vi "Close.vi"(8 "error in (no error)":errorcluster, 11 "RemoteConnection in":refnum<class "RemoteConnection.lvclass">) -> (0 "error out":errorcluster, 3 "RemoteConnection out":refnum<class "RemoteConnection.lvclass">)   [LabVIEW 2013, in "RemoteConnection.lvclass"]
uses:
  RemoteConnection.lvclass
  RemoteConnection.lvclass/RemoteConnection.ctl
  Message/VariantMessage/VariantMessage.lvclass
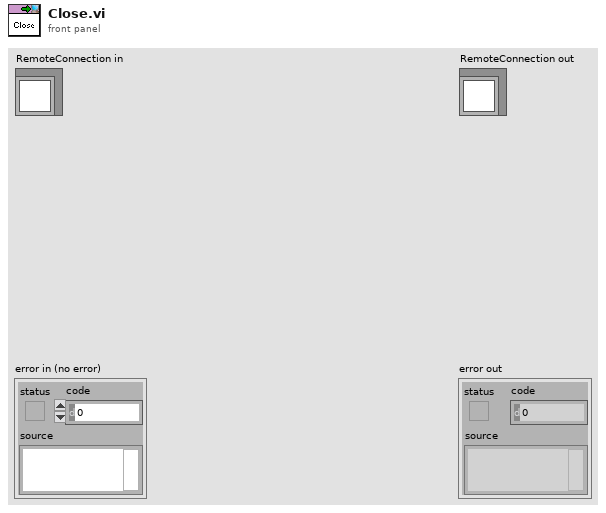
[diagram p1: front panel]
types:
  T1 = typedef "message_queue.ctl" = refnum<queue>
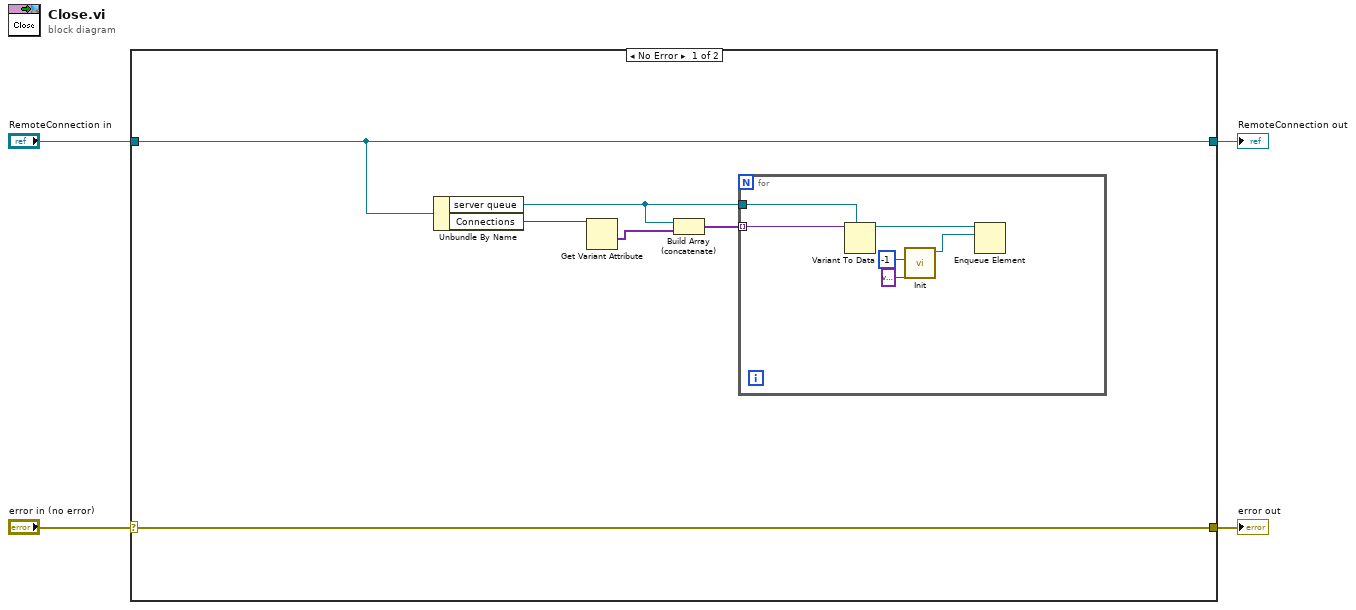
[diagram p0: block diagram]
diagram:
  n1 = case shown="No Error" "error in (no error)" {
    selector: "error in (no error)" -> [w10 w18]
    tunnel: [w10 w18] -> w3
    tunnel: [w9 w17] -> w1
    tunnel: "RemoteConnection in" -> [w9 w17]
    frame No Error {
      n2 = Unbundle By Name(w9) -> ("server queue"=w5:T1, "Connections"=w8:variant)
      n3 = Get Variant Attribute(Variant=w8) -> (values=w7:variant[])  [unwired: 3 in, 3 out]
      n4 = Build Array (concatenate)(w5, w7) -> (w6:variant[])
      n5 = for {
        tunnel: w6 -> [w13] mode=indexing
        tunnel: w5 -> [w12]
        n6 = Variant To Data(type=w12, Variant=w13) -> (data=w11:T1)  [unwired: 1 in, 1 out]
        n7 = call "Init.vi"("Data"=variant, "Type"=-1) -> ("VariantMessage out"=w15:refnum<class "VariantMessage.lvclass">)  [unwired: 8 in, 1 out]
        n8 = Enqueue Element(queue=w11, element=w15) -> ()  [unwired: 2 in, 3 out]
      }
    }
    frame Error {
    }
  }
  "error out" <- w3
  "RemoteConnection out" <- w1
